vi "calculate_correction_m.vi"(0 "grid size for u* and v*":i16=40, 1 "grid size for z*":i16=32, 2 "input file":string, 3 "orientation":enum16{"uv", "uw"}(ring)) -> (6 "Results":string[][](table))   [LabVIEW 2010]
panel:
  out "?":dbl(slide) scale=0.0..100.0 scale format="%.1f"
  out "percent completed":dbl format="%.2f"
  in  "constants":T1={"u'/U"=0.5, "v'/U"=0.4, "w'/U"=0.4, "rho"=0.5, "alpha1"=0.0, "alpha2"=0.0} {"alpha2" format="%.2f"; "alpha1" format="%.2f"; "rho" format="%.2f"; "w'/U" format="%.2f"; "v'/U" format="%.2f"; "u'/U" format="%.2f"}
  in  "u*, v* limits":T2={"u* low"=0.4, "u* high"=1.8, "v* low"=-0.6, "v* high"=0.8} {"v* high" format="%.2f"; "v* low" format="%.2f"; "u* high" format="%.2f"; "u* low" format="%.2f"}
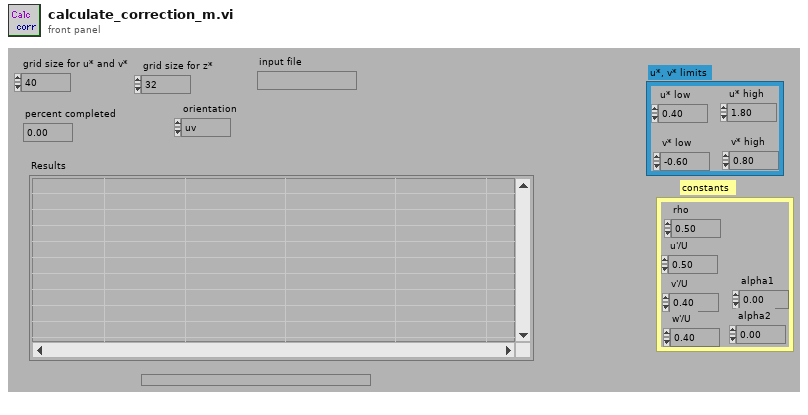
[diagram p1: front panel]
types:
  T1 = cluster{"u'/U":dbl, "v'/U":dbl, "w'/U":dbl, "rho":dbl, "alpha1":dbl, "alpha2":dbl}
  T2 = cluster{"u* low":dbl, "u* high":dbl, "v* low":dbl, "v* high":dbl}
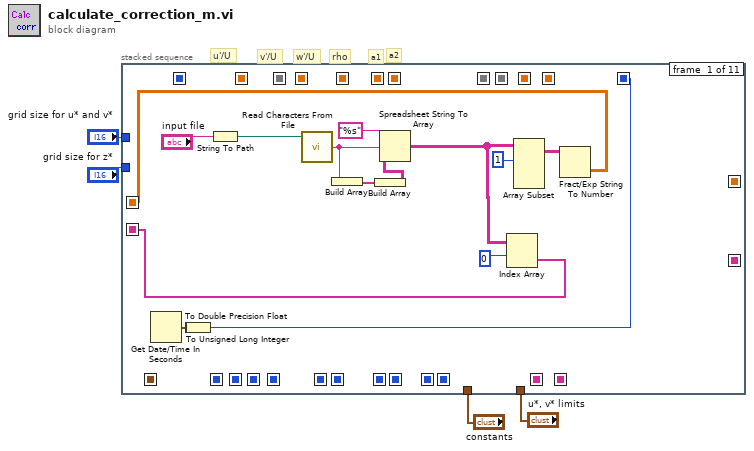
[diagram p0: block diagram]
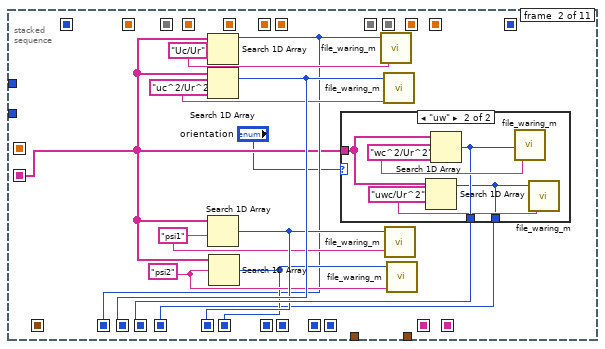
[diagram p2: hidden frame]
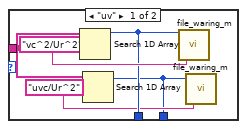
[diagram p3: hidden frame]
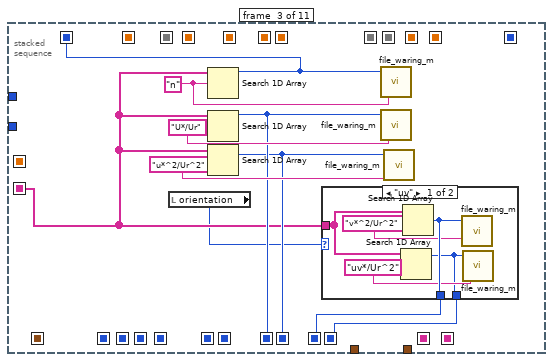
[diagram p4: hidden frame]
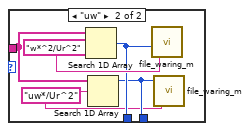
[diagram p5: hidden frame]
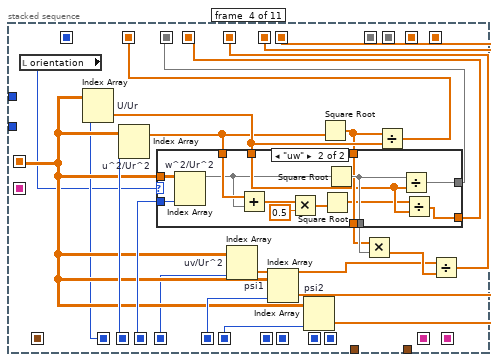
[diagram p6: hidden frame]
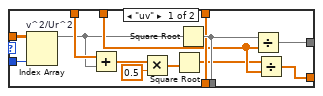
[diagram p7: hidden frame]
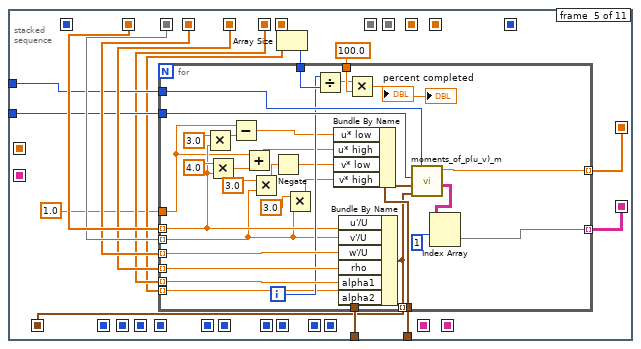
[diagram p8: hidden frame]
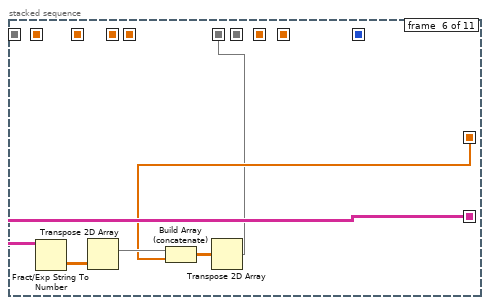
[diagram p9: hidden frame]
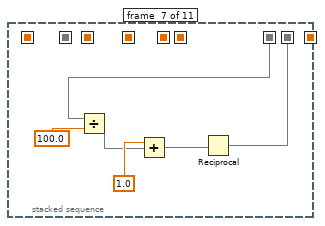
[diagram p10: hidden frame]
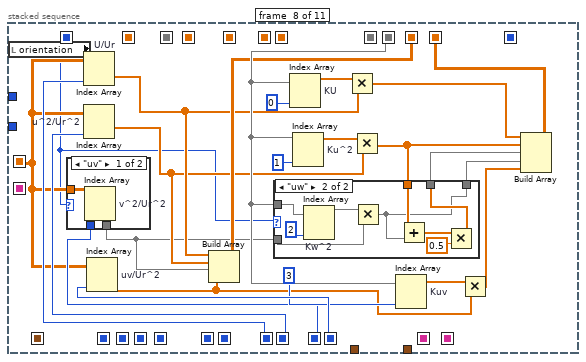
[diagram p11: hidden frame]
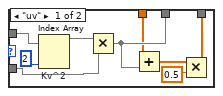
[diagram p12: hidden frame]
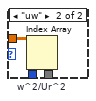
[diagram p13: hidden frame]
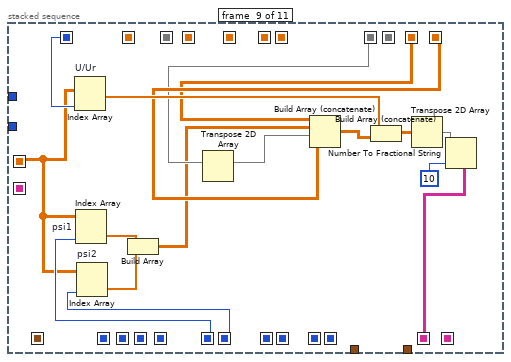
[diagram p14: hidden frame]
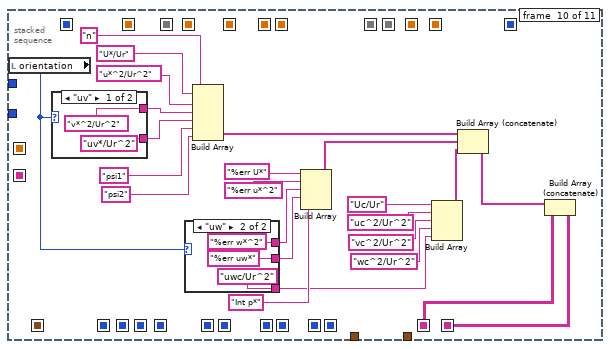
[diagram p15: hidden frame]
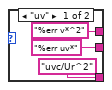
[diagram p16: hidden frame]
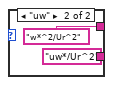
[diagram p17: hidden frame]
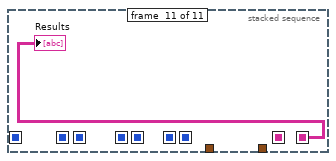
[diagram p18: hidden frame]
diagram:
  # "rho"
  # "a2"
  # "a1"
  # "w'/U"
  # "v'/U"
  # "u'/U"
  n1 = stacked-sequence {
    seq-local: [_ _ _ _ w115 _ _ _ _ _ _] -> [_ _ _ _ _ w163 _ _ _ _ _]
    seq-local: [_ _ _ _ w116 _ _ _ _ _ _] -> [_ _ _ _ _ w159 _ _ _ _ _]
    seq-local: [_ _ _ _ w109 _ _ _ _ _ _] -> [_ _ _ _ _ _ _ _ _ _ _]
    seq-local: [_ _ _ _ _ _ _ _ _ w243 _] -> [_ _ _ _ _ _ _ _ _ _ w269]
    seq-local: [w12 _ _ _ _ _ _ _ _ _ _] -> [_ _ _ w76 _ _ _ w177 w221 _ _]
    seq-local: [_ w31 _ _ _ _ _ _ _ _ _] -> [_ _ _ w82 _ _ _ _ _ _ _]
    seq-local: [_ w29 _ _ _ _ _ _ _ _ _] -> [_ _ _ w81 _ _ _ _ _ _ _]
    seq-local: [_ w28 _ _ _ _ _ _ _ _ _] -> [_ _ _ w80 _ _ _ _ w223 _ _]
    seq-local: [_ _ _ w73 _ _ _ _ _ _ _] -> [_ _ _ _ w123 _ _ _ _ _ _]
    seq-local: [_ _ _ w72 _ _ _ _ _ _ _] -> [_ _ _ _ w122 _ _ _ _ _ _]
    seq-local: [_ _ _ w71 _ _ _ _ _ _ _] -> [_ _ _ _ w121 _ _ _ _ _ _]
    seq-local: [_ _ _ w67 _ _ _ _ _ _ _] -> [_ _ _ _ w120 _ _ _ _ _ _]
    seq-local: [_ _ _ w79 _ _ _ _ _ _ _] -> [_ _ _ _ w112 _ _ _ _ _ _]
    seq-local: [w10 _ _ _ _ _ _ _ _ _ _] -> [_ w22 w46 _ _ _ _ _ _ _ _]
    seq-local: [_ w25 _ _ _ _ _ _ _ _ _] -> [_ _ _ w77 _ _ _ _ w222 _ _]
    seq-local: [_ _ _ w78 _ _ _ _ _ _ _] -> [_ _ _ _ w111 _ _ _ _ _ _]
    seq-local: [w9 _ _ _ _ _ _ _ _ _ _] -> [_ _ _ _ _ _ _ _ _ _ _]
    seq-local: [_ w23 _ _ _ _ _ _ _ _ _] -> [_ _ _ w75 _ _ _ _ _ _ _]
    seq-local: [_ _ w49 _ _ _ _ _ _ _ _] -> [_ _ _ _ _ _ _ w193 _ _ _]
    seq-local: [_ _ w48 _ _ _ _ _ _ _ _] -> [_ _ _ _ _ _ _ w192 _ _ _]
    seq-local: [_ _ w45 _ _ _ _ _ _ _ _] -> [_ _ _ _ _ _ _ w178 _ _ _]
    seq-local: [_ _ w43 _ _ _ _ _ _ _ _] -> [_ _ _ _ _ _ _ w191 _ _ _]
    seq-local: [_ _ _ _ _ w158 _ _ _ _ _] -> [_ _ _ _ _ _ w167 _ w228 _ _]
    seq-local: [_ _ _ _ _ _ w164 _ _ _ _] -> [_ _ _ _ _ _ _ w190 _ _ _]
    seq-local: [_ _ _ _ _ _ _ w176 _ _ _] -> [_ _ _ _ _ _ _ _ w226 _ _]
    seq-local: [_ _ _ _ _ _ _ w175 _ _ _] -> [_ _ _ _ _ _ _ _ w230 _ _]
    seq-local: [_ _ _ _ _ _ _ _ w233 _ _] -> [_ _ _ _ _ _ _ _ _ w237 _]
    seq-local: [_ _ w47 _ _ _ _ _ _ _ _] -> [_ _ _ _ _ _ _ _ w232 _ _]
    seq-local: [_ w20 _ _ _ _ _ _ _ _ _] -> [_ _ _ w66 _ _ _ _ _ _ _]
    tunnel: "grid size for u* and v*" -> [_ _ _ _ w119 _ _ _ _ _ _]
    tunnel: "grid size for z*" -> [_ _ _ _ w118 _ _ _ _ _ _]
    tunnel: "u*, v* limits" -> [_ _ _ _ w117 _ _ _ _ _ _]
    tunnel: "constants" -> [_ _ _ _ w124 _ _ _ _ _ _]
    frame #0 {
      n2 = Get Date/Time In Seconds() -> (seconds since 1Jan1904=w6:timestamp)
      n3 = To Double Precision Float(number=w6) -> (double precision float=w7:dbl)
      n4 = To Unsigned Long Integer(number=w7) -> (unsigned 32bit integer=w9:u32)
      n5 = String To Path(string="input file") -> (path=w5:path)
      n6 = call <vilib>:"Read Characters From File.vi"("file path (dialog if empty)"=w5) -> ("character string"=w15:string)  [unwired: 5 in, 3 out]
      n7 = Build Array(w15) -> (w18:string[])
      n8 = Build Array(w18) -> (w17:string[][])
      n9 = Spreadsheet String To Array(format string="%s", spreadsheet string=w15, array type (2D Dbl)=w17) -> (array=w8:string[][])  [unwired: 1 in]
      n10 = Index Array(array=w8, index (row)=0) -> (element=w10:string[])  [unwired: 1 in]
      n11 = Array Subset(array=w8, index (row)=1) -> (w11:string[][])  [unwired: 3 in]
      n12 = Fract/Exp String To Number(string=w11) -> (number=w12:dbl[][])  [unwired: 3 in, 1 out]
    }
    frame #1 {
      w24 = "Uc/Ur"
      w26 = "psi2"
      w27 = "psi1"
      w30 = "uc^2/Ur^2"
      n13 = Search 1D Array(1D array=w22, element=w24) -> (index of element=w23:i32)  [unwired: 1 in]
      n14 = Search 1D Array(1D array=w22, element=w30) -> (index of element=w31:i32)  [unwired: 1 in]
      n15 = Search 1D Array(1D array=w22, element=w27) -> (index of element=w28:i32)  [unwired: 1 in]
      n16 = Search 1D Array(1D array=w22, element=w26) -> (index of element=w25:i32)  [unwired: 1 in]
      n17 = case shown="\"uw\"" "orientation" {
        tunnel: w22 -> [w34 w38]
        tunnel: [w35 w40] -> w29
        tunnel: [w32 w37] -> w20
        frame "uv" {
          w33 = "uvc/Ur^2"
          w36 = "vc^2/Ur^2"
          n18 = Search 1D Array(1D array=w34, element=w36) -> (index of element=w35:i32)  [unwired: 1 in]
          n19 = Search 1D Array(1D array=w34, element=w33) -> (index of element=w32:i32)  [unwired: 1 in]
          n20 = call "file_waring_m.vi"("item not found"=w36, "index"=w35) -> ()  [unwired: 3 in]
          n21 = call "file_waring_m.vi"("item not found"=w33, "index"=w32) -> ()  [unwired: 3 in]
        }
        frame "uw" {
          w39 = "uwc/Ur^2"
          w41 = "wc^2/Ur^2"
          n22 = Search 1D Array(1D array=w38, element=w39) -> (index of element=w37:i32)  [unwired: 1 in]
          n23 = Search 1D Array(1D array=w38, element=w41) -> (index of element=w40:i32)  [unwired: 1 in]
          n24 = call "file_waring_m.vi"("item not found"=w41, "index"=w40) -> ()  [unwired: 3 in]
          n25 = call "file_waring_m.vi"("item not found"=w39, "index"=w37) -> ()  [unwired: 3 in]
        }
      }
      n26 = call "file_waring_m.vi"("item not found"=w24, "index"=w23) -> ()  [unwired: 3 in]
      n27 = call "file_waring_m.vi"("item not found"=w30, "index"=w31) -> ()  [unwired: 3 in]
      n28 = call "file_waring_m.vi"("item not found"=w27, "index"=w28) -> ()  [unwired: 3 in]
      n29 = call "file_waring_m.vi"("item not found"=w26, "index"=w25) -> ()  [unwired: 3 in]
    }
    frame #2 {
      w42 = "n"
      w50 = "U*/Ur"
      w51 = "u*^2/Ur^2"
      n30 = local read "orientation"() -> (w44:enum16{"uv", "uw"})
      n31 = Search 1D Array(1D array=w46, element=w42) -> (index of element=w47:i32)  [unwired: 1 in]
      n32 = Search 1D Array(1D array=w46, element=w50) -> (index of element=w49:i32)  [unwired: 1 in]
      n33 = Search 1D Array(1D array=w46, element=w51) -> (index of element=w48:i32)  [unwired: 1 in]
      n34 = case shown="\"uv\"" w44 {
        tunnel: w46 -> [w52 w58]
        tunnel: [w56 w60] -> w45
        tunnel: [w53 w59] -> w43
        frame "uv" {
          w54 = "uv*/Ur^2"
          w55 = "v*^2/Ur^2"
          n35 = Search 1D Array(1D array=w52, element=w54) -> (index of element=w53:i32)  [unwired: 1 in]
          n36 = Search 1D Array(1D array=w52, element=w55) -> (index of element=w56:i32)  [unwired: 1 in]
          n37 = call "file_waring_m.vi"("item not found"=w55, "index"=w56) -> ()  [unwired: 3 in]
          n38 = call "file_waring_m.vi"("item not found"=w54, "index"=w53) -> ()  [unwired: 3 in]
        }
        frame "uw" {
          w57 = "uw*/Ur^2"
          w61 = "w*^2/Ur^2"
          n39 = Search 1D Array(1D array=w58, element=w61) -> (index of element=w60:i32)  [unwired: 1 in]
          n40 = Search 1D Array(1D array=w58, element=w57) -> (index of element=w59:i32)  [unwired: 1 in]
          n41 = call "file_waring_m.vi"("item not found"=w61, "index"=w60) -> ()  [unwired: 3 in]
          n42 = call "file_waring_m.vi"("item not found"=w57, "index"=w59) -> ()  [unwired: 3 in]
        }
      }
      n43 = call "file_waring_m.vi"("item not found"=w42, "index"=w47) -> ()  [unwired: 3 in]
      n44 = call "file_waring_m.vi"("item not found"=w50, "index"=w49) -> ()  [unwired: 3 in]
      n45 = call "file_waring_m.vi"("item not found"=w51, "index"=w48) -> ()  [unwired: 3 in]
    }
    frame #3 {
      n46 = local read "orientation"() -> (w65:enum16{"uv", "uw"})
      n47 = Index Array "U/Ur"(array=w76, index (col)=w75) -> (element=w74:dbl[])  [unwired: 1 in]
      n48 = Index Array "u^2/Ur^2"(array=w76, index (col)=w82) -> (element=w62:dbl[])  [unwired: 1 in]
      n49 = Index Array "uv/Ur^2"(array=w76, index (col)=w66) -> (element=w68:dbl[])  [unwired: 1 in]
      n50 = Index Array "psi1"(array=w76, index (col)=w80) -> (element=w79:dbl[])  [unwired: 1 in]
      n51 = Index Array "psi2"(array=w76, index (col)=w77) -> (element=w78:dbl[])  [unwired: 1 in]
      n52 = Square Root(x=w62) -> (sqrt(x)=w64:dbl[])
      n53 = case shown="\"uw\"" w65 {
        tunnel: [w95 w108] -> w70
        tunnel: [w90 w96] -> w71
        tunnel: [w94 w97] -> w72
        tunnel: w74 -> [w89 w104]
        tunnel: w76 -> [w93 w107]
        tunnel: w81 -> [w92 w106]
        tunnel: w64 -> [w91 w105]
        tunnel: [w91 w105] -> w63
        tunnel: w62 -> [w87 w102]
        frame "uv" {
          n54 = Index Array "v^2/Ur^2"(array=w93, index (col)=w92) -> (element=w86:dbl[])  [unwired: 1 in]
          n55 = Add(x=w87, y=w86) -> (x+y=w85:dbl[])
          n56 = Multiply(x=w85, y=0.5) -> (x*y=w83:dbl[])
          n57 = Square Root(x=w83) -> (sqrt(x)=w88:dbl[])
          n58 = Square Root(x=w86) -> (sqrt(x)=w95:dbl[])
          n59 = Divide(x=w95, y=w89) -> (x/y=w94:dbl[])
          n60 = Divide(x=w88, y=w89) -> (x/y=w90:dbl[])
        }
        frame "uw" {
          n61 = Index Array "w^2/Ur^2"(array=w107, index (col)=w106) -> (element=w101:dbl[])  [unwired: 1 in]
          n62 = Add(x=w102, y=w101) -> (x+y=w100:dbl[])
          n63 = Multiply(x=w100, y=0.5) -> (x*y=w98:dbl[])
          n64 = Square Root(x=w98) -> (sqrt(x)=w103:dbl[])
          n65 = Square Root(x=w101) -> (sqrt(x)=w108:dbl[])
          n66 = Divide(x=w108, y=w104) -> (x/y=w97:dbl[])
          n67 = Divide(x=w103, y=w104) -> (x/y=w96:dbl[])
        }
      }
      n68 = Multiply(x=w63, y=w70) -> (x*y=w69:dbl[])
      n69 = Divide(x=w64, y=w74) -> (x/y=w73:dbl[])
      n70 = Divide(x=w68, y=w69) -> (x/y=w67:dbl[])
    }
    frame #4 {
      n71 = Array Size(array=w111) -> (size(s)=w114:i32)
      n72 = for {
        tunnel: w124 -> [w157]
        tunnel: 1.0 -> [w126]
        tunnel: w123 -> [w137] mode=indexing
        tunnel: w122 -> [w134] mode=indexing
        tunnel: w121 -> [w156] mode=indexing
        tunnel: w120 -> [w155] mode=indexing
        tunnel: w112 -> [w154] mode=indexing
        tunnel: w119 -> [w153]
        tunnel: w118 -> [w152]
        tunnel: w117 -> [w151]
        tunnel: [w147] -> w116 mode=indexing
        tunnel: [w146] -> w115 mode=indexing
        tunnel: [w145] -> w109 mode=indexing
        tunnel: w114 -> [w144]
        tunnel: 100.0 -> [w141]
        tunnel: w111 -> [w140] mode=indexing
        i -> [w143]
        n73 = Multiply(x=3.0, y=w137) -> (x*y=w127:dbl)
        n74 = Multiply(x=4.0, y=w137) -> (x*y=w130:dbl)
        n75 = Subtract(x=w126, y=w127) -> (x-y=w128:dbl)
        n76 = Add(x=w126, y=w130) -> (x+y=w129:dbl)
        n77 = Multiply(x=3.0, y=w134) -> (x*y=w133:dbl)
        n78 = Negate(x=w133) -> (-x=w131:dbl)
        n79 = Multiply(x=3.0, y=w134) -> (x*y=w132:dbl)
        n80 = Divide(x=w143, y=w144) -> (x/y=w125:dbl)
        n81 = Bundle By Name(cluster=w151, "u* low"=w128, "u* high"=w129, "v* low"=w131, "v* high"=w132) -> (w150:T2)
        n82 = Bundle By Name(cluster=w157, "u'/U"=w137, "v'/U"=w134, "w'/U"=w156, "rho"=w155, "alpha1"=w154, "alpha2"=w140) -> (w145:T1)
        n83 = Multiply(x=w125, y=w141) -> (x*y=→"percent completed" →"?":dbl)
        n84 = call "moments_of_p(u_v)_m.vi"("constants"=w145, "u*, v* limits"=w150, "grid size for z*"=w152, "grid size for u* and v*"=w153) -> ("Results table"=w148:string[][], "Volume under p(u*,v*)"=w147:dbl)  [unwired: 6 in]
        n85 = Index Array(array=w148, index (row)=1) -> (element=w146:string[])  [unwired: 1 in]
      }
    }
    frame #5 {
      n86 = Fract/Exp String To Number(string=w163) -> (number=w160:dbl[][])  [unwired: 3 in, 1 out]
      n87 = Transpose 2D Array(2D array=w160) -> (transposed array=w162:dbl[][])
      n88 = Build Array (concatenate)(w162, w159) -> (w161:dbl[][])
      n89 = Transpose 2D Array(2D array=w161) -> (transposed array=w158:dbl[][])
    }
    frame #6 {
      n90 = Divide(x=w167, y=100.0) -> (x/y=w166:dbl[][])
      n91 = Add(x=1.0, y=w166) -> (x+y=w165:dbl[][])
      n92 = Reciprocal(x=w165) -> (1/x=w164:dbl[][])
    }
    frame #7 {
      n93 = local read "orientation"() -> (w172:enum16{"uv", "uw"})
      n94 = case shown="\"uv\"" w172 {
        tunnel: w177 -> [w214 w217]
        tunnel: w178 -> [w213 w216]
        tunnel: [w212 w215] -> w170
        frame "uv" {
          n95 = Index Array "v^2/Ur^2"(array=w214, index (col)=w213) -> (element=w212:dbl[])  [unwired: 1 in]
        }
        frame "uw" {
          n96 = Index Array "w^2/Ur^2"(array=w217, index (col)=w216) -> (element=w215:dbl[])  [unwired: 1 in]
        }
      }
      n97 = Index Array "U/Ur"(array=w177, index (col)=w193) -> (element=w174:dbl[])  [unwired: 1 in]
      n98 = Index Array "u^2/Ur^2"(array=w177, index (col)=w192) -> (element=w173:dbl[])  [unwired: 1 in]
      n99 = Index Array "uv/Ur^2"(array=w177, index (col)=w191) -> (element=w179:dbl[])  [unwired: 1 in]
      n100 = Build Array(w174, w173, w170, w179) -> (w176:dbl[][])
      n101 = Index Array "KU"(array=w190, index (col)=0) -> (element=w184:dbl[])  [unwired: 1 in]
      n102 = Index Array "Ku^2"(array=w190, index (col)=1) -> (element=w185:dbl[])  [unwired: 1 in]
      n103 = Multiply(x=w184, y=w174) -> (x*y=w183:dbl[])
      n104 = Multiply(x=w185, y=w173) -> (x*y=w182:dbl[])
      n105 = case shown="\"uw\"" w172 {
        tunnel: [w202 w204] -> w181
        tunnel: w182 -> [w201 w211]
        tunnel: w190 -> [w196 w206]
        tunnel: [w195 w203] -> w171
        tunnel: w170 -> [w194 w205]
        frame "uv" {
          n106 = Index Array "Kv^2"(array=w196, index (col)=2) -> (element=w198:dbl[])  [unwired: 1 in]
          n107 = Multiply(x=w198, y=w194) -> (x*y=w202:dbl[])
          n108 = Add(x=w201, y=w202) -> (x+y=w199:dbl[])
          n109 = Multiply(x=w199, y=0.5) -> (x*y=w195:dbl[])
        }
        frame "uw" {
          n110 = Index Array "Kw^2"(array=w206, index (col)=2) -> (element=w208:dbl[])  [unwired: 1 in]
          n111 = Multiply(x=w208, y=w205) -> (x*y=w203:dbl[])
          n112 = Add(x=w211, y=w203) -> (x+y=w209:dbl[])
          n113 = Multiply(x=w209, y=0.5) -> (x*y=w204:dbl[])
        }
      }
      n114 = Index Array "Kuv"(array=w190, index (col)=3) -> (element=w186:dbl[])  [unwired: 1 in]
      n115 = Multiply(x=w186, y=w179) -> (x*y=w180:dbl[])
      n116 = Build Array(w183, w182, w181, w171, w180) -> (w175:dbl[][])
    }
    frame #8 {
      n117 = Index Array "U/Ur"(array=w221, index (col)=w232) -> (element=w231:dbl[])  [unwired: 1 in]
      n118 = Index Array "psi1"(array=w221, index (col)=w223) -> (element=w220:dbl[])  [unwired: 1 in]
      n119 = Index Array "psi2"(array=w221, index (col)=w222) -> (element=w219:dbl[])  [unwired: 1 in]
      n120 = Build Array(w220, w219) -> (w218:dbl[][])
      n121 = Transpose 2D Array(2D array=w228) -> (transposed array=w227:dbl[][])
      n122 = Build Array (concatenate)(w226, w218, w227, w230) -> (w229:dbl[][])
      n123 = Build Array (concatenate)(w231, w229) -> (w225:dbl[][])
      n124 = Transpose 2D Array(2D array=w225) -> (transposed array=w224:dbl[][])
      n125 = Number To Fractional String(number=w224, precision (6)=10) -> (F-format string=w233:string[][])  [unwired: 2 in]
    }
    frame #9 {
      n126 = local read "orientation"() -> (w238:enum16{"uv", "uw"})
      n127 = case shown="\"uv\"" w238 {
        tunnel: ["v*^2/Ur^2" "w*^2/Ur^2"] -> w240
        tunnel: ["uv*/Ur^2" "uw*/Ur^2"] -> w239
        frame "uv" {
        }
        frame "uw" {
        }
      }
      n128 = case shown="\"uw\"" w238 {
        tunnel: ["%err uv*" "%err uw*"] -> w253
        tunnel: ["%err v*^2" "%err w*^2"] -> w254
        tunnel: ["uvc/Ur^2" "uwc/Ur^2"] -> w235
        frame "uv" {
        }
        frame "uw" {
        }
      }
      n129 = Build Array("n", "U*/Ur", "u*^2/Ur^2", w240, w239, "psi1", "psi2") -> (w247:string[])
      n130 = Build Array("%err U*", "%err u*^2", w254, w253, "Int p*") -> (w246:string[])
      n131 = Build Array("Uc/Ur", "uc^2/Ur^2", "vc^2/Ur^2", "wc^2/Ur^2", w235) -> (w245:string[])
      n132 = Build Array (concatenate)(w247, w246, w245) -> (w244:string[])
      n133 = Build Array (concatenate)(w244, w237) -> (w243:string[][])
    }
    frame #10 {
      "Results" <- w269
    }
  }
